vi "Z-ControllerInterFace.vi"() -> (0 "motorref":refnum<k7>)   [LabVIEW 2015]
panel:
  in  "MG17Motor":refnum<k7>(container)
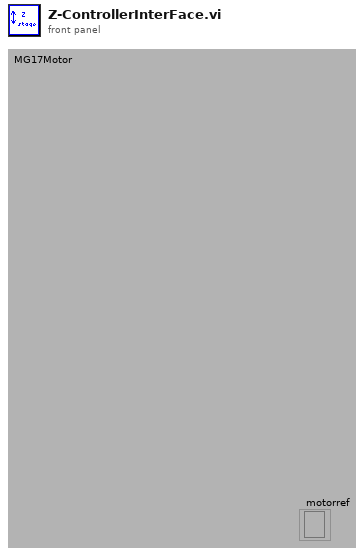
[diagram p1: front panel]
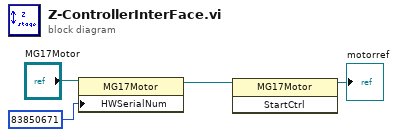
[diagram p0: block diagram]
diagram:
  n1 = property class="MG17Motor"(reference="MG17Motor", "HWSerialNum"=83850671) -> (reference out=w2:refnum<k7>)  [unwired: 1 in, 1 out]
  n2 = invoke class="MG17Motor" method="StartCtrl"(reference=w2) -> (reference out=→"motorref":refnum<k7>)  [unwired: 2 in, 2 out]
